vi "Handle MissionOp Loiter.vi"(8 "error in (no error)":errorcluster, 11 "RDS Mission Controller Actor in":refnum<class "RDS Mission Controller Actor.lvclass">) -> (0 "error out":errorcluster, 3 "RDS Mission Controller Actor out":refnum<class "RDS Mission Controller Actor.lvclass">)   [LabVIEW 2015, in "RDS Mission Controller Actor.lvlib" / "RDS Mission Controller Actor.lvclass"]
uses:
  RDS Mission Controller Actor.lvclass
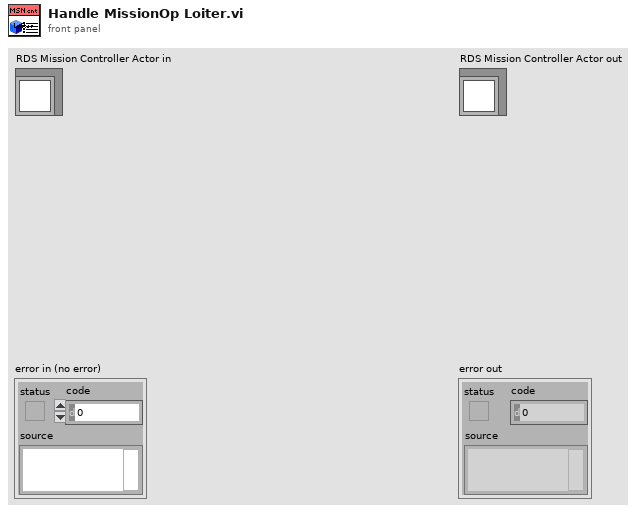
[diagram p1: front panel]
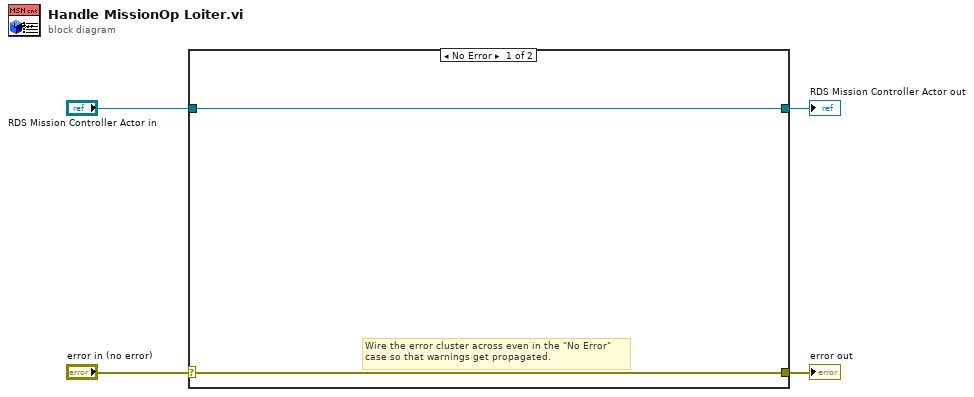
[diagram p0: block diagram]
diagram:
  n1 = case shown="No Error" "error in (no error)" {
    selector: "error in (no error)" -> [w5 w8]
    tunnel: [w5 w8] -> w3
    tunnel: [w6 w7] -> w1
    tunnel: "RDS Mission Controller Actor in" -> [w6 w7]
    frame No Error {
      # "Wire the error cluster across even in the \"No Error\"\ncase so that warnings get propagated."
    }
    frame Error {
    }
  }
  "error out" <- w3
  "RDS Mission Controller Actor out" <- w1
